vi "Login_Test.vi"() -> ()   [LabVIEW 2014]
panel:
  in  "Login":T1
  in  "정지":bool
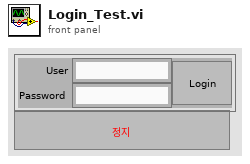
[diagram p1: front panel]
types:
  T1 = cluster{"User":string, "Password":string, "Login":bool}
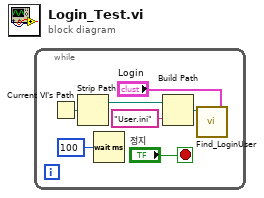
[diagram p0: block diagram]
diagram:
  n1 = while {
    stop <- "정지" stop-if-true
    n2 = Current VI's Path() -> (path=w4:path)
    n3 = Strip Path(path=w4) -> (stripped path=w3:path)  [unwired: 1 out]
    n4 = Wait (ms)(milliseconds to wait=u32 100 ("대기 시간(ms)")) -> ()  [unwired: 1 out]
    n5 = Build Path(base path=w3, name or relative path="User.ini" ("이름 또는 상대 경로")) -> (appended path=w1:path)
    n6 = call "Find_LoginUser.vi"("Login"="Login", "Root of UserList File"=w1) -> ()  [unwired: 5 in, 1 out]
  }
